vi "LL_GET Object.vi"(8 "error in (no error)":errorcluster, 9 "Bucket":string, 10 "Path and query string":string="/", 11 "Headers":T2[](array[typedef])) -> (0 "error out":errorcluster, 1 "Call Result":T1, 2 "Response body":string, 3 "Response header":string)   [LabVIEW 2011, in "LV Interface for Amazon S3.lvlib"]
doc: "This core implementation of the GET operation retrieves objects from Amazon S3. You have direct access to HTTP headers, can set the query string at the end of the path, so you can use this VI to implement special requests or API calls not present in this toolkit."
uses:
  LV Interface for Amazon S3.lvlib
  Typedefs/AMZ_S3_HTTP Header-Value pair.ctl
  Typedefs/AMZ_S3_Call Results.ctl
  <vilib>/regexp/Match Regular Expression.xnode
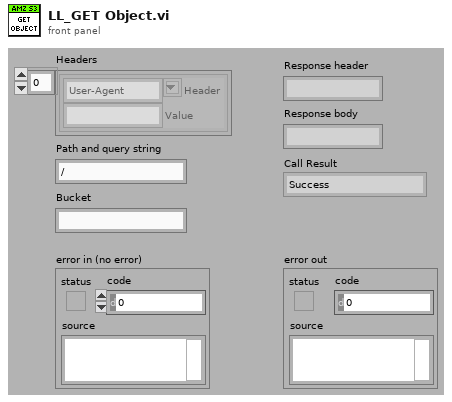
[diagram p1: front panel]
types:
  T1 = typedef "LV Interface for Amazon S3.lvlib/AMZ_S3_Call Results.ctl" = enum16{"Success", "UndefinedError", "AccessDenied", "AccountProblem", "AmbiguousGrantByEmailAddress", "BadDigest", "BucketAlreadyExists", "BucketAlreadyOwnedByYou", "BucketNotEmpty", "CredentialsNotSupported", "CrossLocationLoggingProhibited", "EntityTooSmall", "EntityTooLarge", "ExpiredToken", "IllegalVersioningConfigurationException", "IncompleteBody", "IncorrectNumberOfFilesInPostRequest", "InlineDataTooLarge", "InternalError", "InvalidAccessKeyId", "InvalidAddressingHeader", "InvalidArgument", "InvalidBucketName", "InvalidDigest", "InvalidLocationConstraint", "InvalidPart", "InvalidPartOrder", "InvalidPayer", "InvalidPolicyDocument", "InvalidRange", "InvalidSecurity", "InvalidSOAPRequest", "InvalidStorageClass", "InvalidTargetBucketForLogging", "InvalidToken", "InvalidURI", "KeyTooLong", "MalformedACLError", "MalformedPOSTRequest", "MalformedXML", "MaxMessageLengthExceeded", "MaxPostPreDataLengthExceededError", "MetadataTooLarge", "MethodNotAllowed", "MissingAttachment", "MissingContentLength", "MissingRequestBodyError", "MissingSecurityElement", "MissingSecurityHeader", "NoLoggingStatusForKey", "NoSuchBucket", "NoSuchKey", "NoSuchUpload", "NoSuchVersion", "NotImplemented", "NotSignedUp", "OperationAborted", "PermanentRedirect", "PreconditionFailed", "Redirect", "RequestIsNotMultiPartContent", "RequestTimeout", "RequestTimeTooSkewed", "RequestTorrentOfBucketError", "SignatureDoesNotMatch", "SlowDown", "TemporaryRedirect", "TokenRefreshRequired", "TooManyBuckets", "UnexpectedContent", "UnresolvableGrantByEmailAddress", "UserKeyMustBeSpecified", "LabVIEWError"}
  T2 = typedef "LV Interface for Amazon S3.lvlib/AMZ_S3_HTTP Header-Value pair.ctl" = cluster{"Header":string, "Value":string}
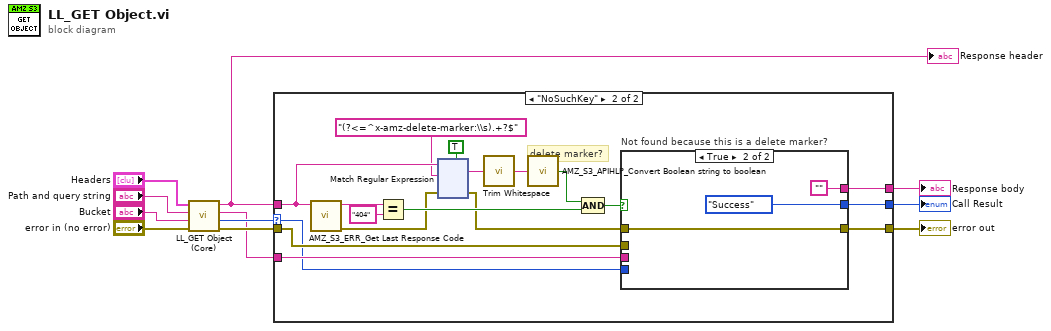
[diagram p0: block diagram]
diagram:
  n1 = call "LL_GET Object (Core).vi"("error in (no error)"="error in (no error)", "Bucket"="Bucket", "Path and query string"="Path and query string", "Headers"="Headers") -> ("error out"=w10:errorcluster, "Call Result"=w11:T1, "Response body"=w2:string, "Response header"=w9:string)  [unwired: 4 in]
  "Response header" <- w9
  n2 = case shown="\"NoSuchKey\"" w11 {
    selector: w11 -> [w13 w16]
    tunnel: w9 -> [_ w30]
    tunnel: w10 -> [w14 w22]
    tunnel: [w14 w15] -> w3
    tunnel: [w13 w19] -> w4
    tunnel: w2 -> [w12 w17]
    tunnel: [w12 w18] -> w1
    frame Default {
    }
    frame "NoSuchKey" {
      # "delete marker?"
      n3 = call "AMZ_S3_ERR_Get Last Response Code.vi"("Response header"=w30) -> ("error out"=w21:errorcluster, "Response code (last)"=w32:string)  [unwired: 9 in]
      n4 = Equal?(x=w32, y="404" ("x")) -> (x = y?=w24:bool)
      n5 = xnode "Match Regular Expression"("input string"=w30, "regular expression"="(?<=^x-amz-delete-marker:\\s).+?$", "error in"=w21, "multiline? (F)"=TRUE) -> ("whole match"=w27:string, "error out"=w20:errorcluster)  [unwired: 2 in, 3 out]
      n6 = call <vilib>:"Trim Whitespace.vi"("string"=w27) -> ("trimmed string"=w26:string)  [unwired: 1 in]
      n7 = call "AMZ_S3_APIHLP_Convert Boolean string to boolean.vi"("Boolean string in"=w26) -> ("Boolean out"=w25:bool)  [unwired: 4 in]
      n8 = Compound Arithmetic op=AND(w25, w24) -> (w23:bool)
      n9 = case "Not found because this is a delete marker?" shown="True" w23 {
        tunnel: w22 -> [w33 _]
        tunnel: w20 -> [_ w36]
        tunnel: [w34 AMZ_S3_Call_Results."Success" ("Call Result")] -> w19
        tunnel: [w35 ""] -> w18
        tunnel: w17 -> [w35 _]
        tunnel: w16 -> [w34 _]
        tunnel: [w33 w36] -> w15
        frame False {
        }
        frame True {
        }
      }
    }
  }
  "Response body" <- w1
  "Call Result" <- w4
  "error out" <- w3
